vi "stacked_Secuence.vi"() -> ()   [LabVIEW 2020]
panel:
  out "Tank 4":u8(slide) scale=0.0..100.0
  out "Tank 3":u8(slide) scale=0.0..100.0
  out "Tank 2":u8(slide) scale=0.0..100.0
  out "Tank":u8(slide) scale=0.0..100.0
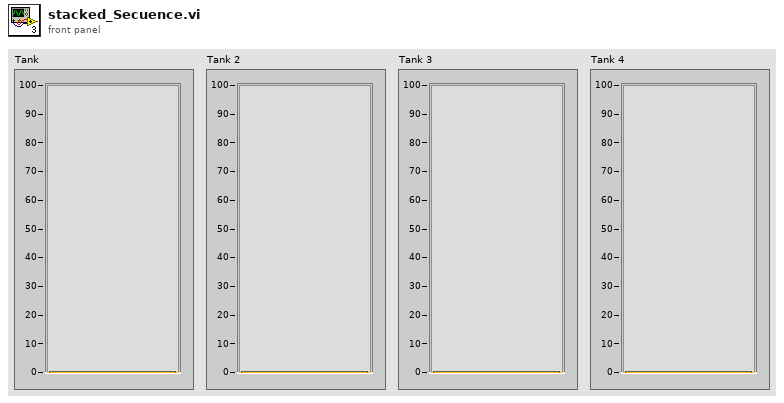
[diagram p1: front panel]
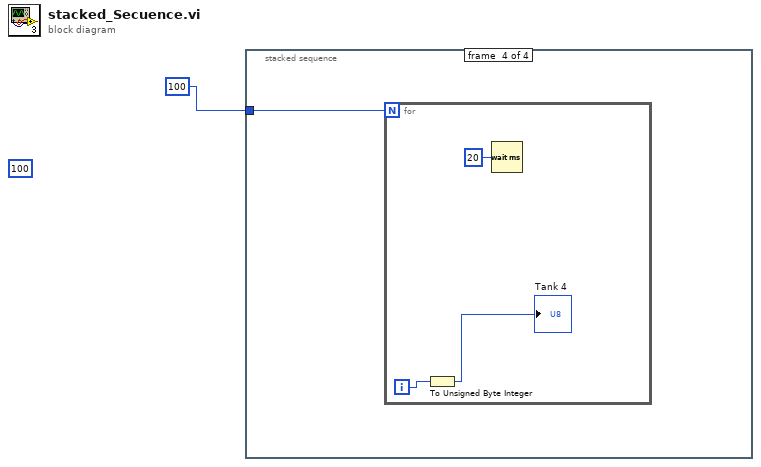
[diagram p0: block diagram]
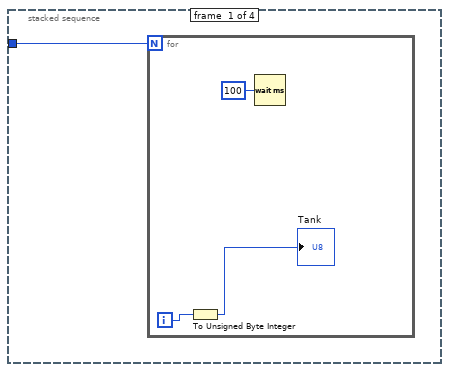
[diagram p2: hidden frame]
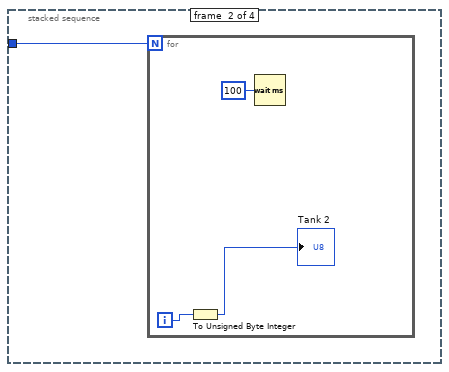
[diagram p3: hidden frame]
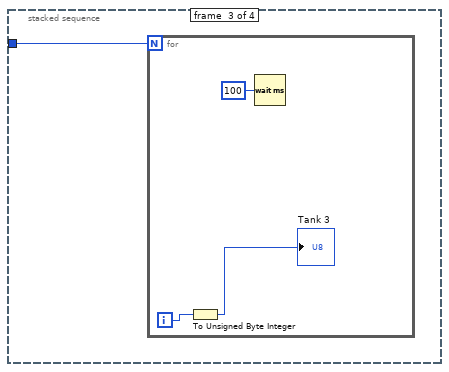
[diagram p4: hidden frame]
diagram:
  (unwired) 100
  n1 = stacked-sequence {
    tunnel: 100 -> [w2 w6 w10 w14]
    frame #0 {
      n2 = for {
        N: w2 -> [_]
        i -> [w5]
        n3 = To Unsigned Byte Integer(number=w5) -> (unsigned 8bit integer=→"Tank":u8)
        n4 = Wait (ms)(milliseconds to wait=u32 100) -> ()  [unwired: 1 out]
      }
    }
    frame #1 {
      n5 = for {
        N: w6 -> [_]
        i -> [w9]
        n6 = To Unsigned Byte Integer(number=w9) -> (unsigned 8bit integer=→"Tank 2":u8)
        n7 = Wait (ms)(milliseconds to wait=u32 100) -> ()  [unwired: 1 out]
      }
    }
    frame #2 {
      n8 = for {
        N: w10 -> [_]
        i -> [w13]
        n9 = To Unsigned Byte Integer(number=w13) -> (unsigned 8bit integer=→"Tank 3":u8)
        n10 = Wait (ms)(milliseconds to wait=u32 100) -> ()  [unwired: 1 out]
      }
    }
    frame #3 {
      n11 = for {
        N: w14 -> [_]
        i -> [w17]
        n12 = To Unsigned Byte Integer(number=w17) -> (unsigned 8bit integer=→"Tank 4":u8)
        n13 = Wait (ms)(milliseconds to wait=u32 20) -> ()  [unwired: 1 out]
      }
    }
  }
